vi "Refresh by Name.vi"(6 "TreeControl in":refnum<vi>, 7 "Data Cluster In":T1={"Project"=refnum, "Current Selection"={"Library"=refnum, "VI"=refnum}, "Module ID"=-1, "Tree Selection"=""}, 8 "error in":errorcluster, 11 "Module Name":string) -> (0 "error out":errorcluster, 5 "Data Cluster Out":T1={"Project"=refnum, "Current Selection"={"Library"=refnum, "VI"=refnum}, "Module ID"=-1, "Tree Selection"=""})   [LabVIEW 2020, in "Panther Dashboard.lvlib"]
doc: "Gets the Singleton and Cloneable references and creates a list of each type of DQMH Modules"
uses:
  Panther Dashboard.lvlib
  Module Data--cluster.ctl
  Class/Project/Project.lvclass
  Class/Library/Library.lvclass
  C:/GitClones/PantherDashboard/src/LabVIEW/Panther Dashboard/Class/LabVIEWItem/LabVIEWItem.lvclass
  Class/VI/VI.lvclass
  Class/Project/Project.lvclass/Project.ctl
  Class/LabVIEWItem/LabVIEWItem.lvclass/LabVIEWItem.ctl
  Class/LabVIEWItem/Item Type--enum.ctl
  Class/Library/Library.lvclass/Library.ctl
  Class/Library/Write VIs MAP.vi
  Class/LabVIEWItem/Read Item Name.vi
  Class/Project/Write Libraries.vi
  Class/Project/Read Libraries.vi
  Class/LabVIEWItem/Read Item Tag.vi
  Class/Project/Read Main App Inst Ref.vi
  Class/LabVIEWItem/LabVIEWItem.lvclass
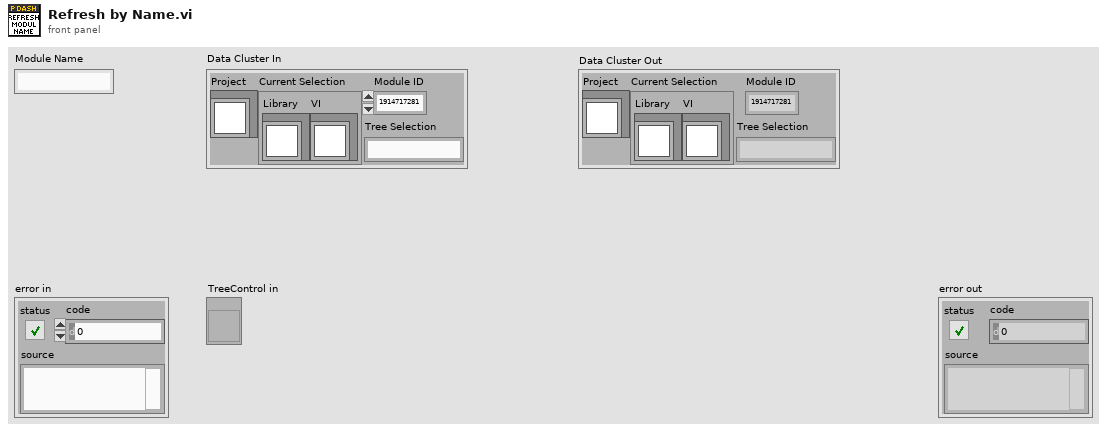
[diagram p1: front panel]
types:
  T1 = typedef "Panther Dashboard.lvlib/Module Data--cluster.ctl" = cluster{"Project":refnum<class "Project.lvclass">, "Current Selection":cluster{"Library":refnum<class "Library.lvclass">, "VI":refnum<class "VI.lvclass">}, "Module ID":i32, "Tree Selection":string}
  T2 = typedef "Panther Dashboard.lvlib/LabVIEWItem.lvclass/Item Type--enum.ctl" = enum16{"Requests", "Broadcasts", "Request and Wait for Reply", "Round Trip", "» Public API VIs", "» Constant VIs", "» Error VIs", "Module", "Project", "No Drag Selection"}
  T3 = typedef "Tree Map.lvlib/Tree Map Data.ctl" = map{string, cluster{"Child Paths Set":set{string}, "Name":string, "Data":string, "Attributes":map{string, string}}}
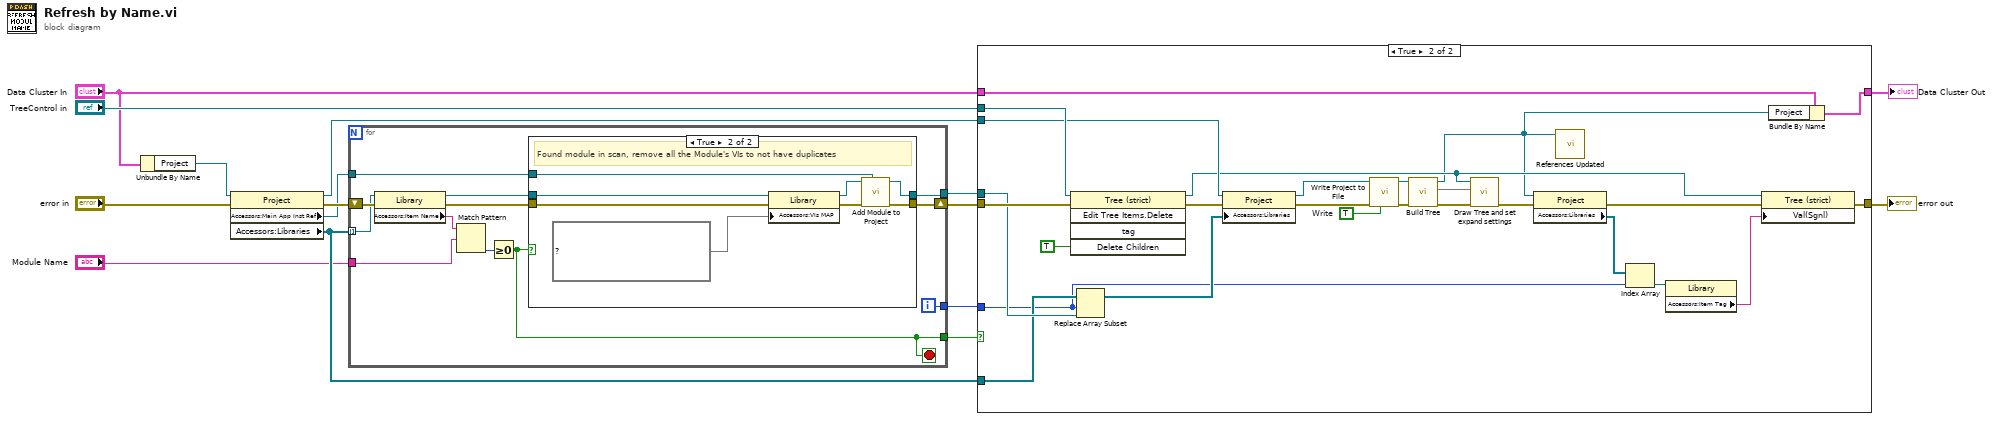
[diagram p0: block diagram]
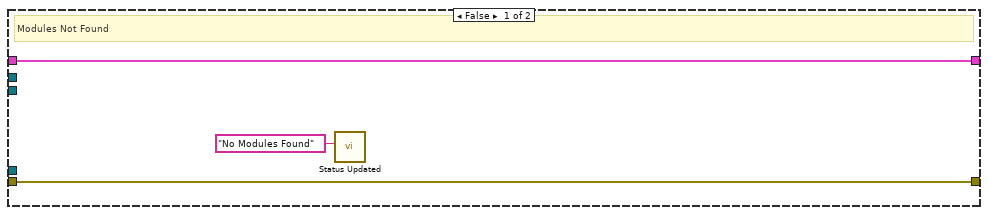
[diagram p2: hidden frame]
diagram:
  n1 = Unbundle By Name("Data Cluster In") -> ("Project"=w8:refnum<class "Project.lvclass">)
  n2 = property class="Project"(reference=w8, error in="error in") -> (reference out=w7:refnum<class "Project.lvclass">, error out=w15:errorcluster, "Accessors:Main App Inst Ref"=w3:refnum<vi>, "Accessors:Libraries"=w4:refnum<class "Library.lvclass">[])
  n3 = for {
    tunnel: w4 -> [w24] mode=indexing
    tunnel: [w23] -> w6
    shift-right: [w25] -> w13
    shift-left: w15 -> [w27]
    tunnel: [w20] -> w5
    tunnel: w3 -> [w21]
    tunnel: "Module Name" -> [w18]
    tunnel: [w16] -> w1
    i -> [w23]
    stop <- w16 stop-if-true
    n4 = property class="Library"(reference=w24, error in=w27) -> (reference out=w22:refnum<class "Library.lvclass">, error out=w26:errorcluster, "Accessors:Item Name"=w19:string)
    n5 = Match Pattern(string=w19, regular expression=w18) -> (offset past match=w17:i32)  [unwired: 1 in, 3 out]
    n6 = Greater Or Equal To 0?(x=w17) -> (x >= 0?=w16:bool)
    n7 = case shown="True" w16 {
      tunnel: w26 -> [w29 w37]
      tunnel: [w29 w36] -> w25
      tunnel: w22 -> [w28 w32]
      tunnel: w21 -> [_ w34]
      tunnel: [w28 w33] -> w20
      frame False {
        # "Current module has different Tag"
      }
      frame True {
        # "Found module in scan, remove all the Module's VIs to not have duplicates"
        n8 = property class="Library"(reference=w32, error in=w37, "Accessors:VIs MAP"=map{T2, refnum<class "VI.lvclass">[]} {} ("VIs MAP")) -> (reference out=w31:refnum<class "Library.lvclass">, error out=w35:errorcluster)
        n9 = call "Add Module to Project.vi"("App Ref"=w34, "error in"=w35, "Library In"=w31) -> ("error out"=w36:errorcluster, "Library Out"=w33:refnum<class "Library.lvclass">)  [unwired: 7 in]
      }
    }
  }
  n10 = case shown="True" w1 {
    tunnel: w13 -> [w40 w66]
    tunnel: [w40 w63] -> w12
    tunnel: "TreeControl in" -> [_ w58]
    tunnel: "Data Cluster In" -> [w39 w55]
    tunnel: [w39 w54] -> w9
    tunnel: w7 -> [_ w53]
    tunnel: w6 -> [_ w44]
    tunnel: w5 -> [_ w49]
    tunnel: w4 -> [_ w46]
    frame False {
      # "Modules Not Found"
      n11 = call "Status Updated.vi"("Status"="No Modules Found") -> ()  [unwired: 10 in, 1 out]
    }
    frame True {
      w56 = TRUE  # Write
      n12 = invoke class="Tree (strict)" method="Edit Tree Items.Delete"(reference=w58, error in=w66, "Delete Children"=TRUE ("Delete Children?")) -> (reference out=w48:refnum<vi>, error out=w65:errorcluster)  [unwired: 2 in, 3 out]
      n13 = Replace Array Subset "Replace Array Subset"(array=w46, new element=w49, index=w44) -> (w47:refnum<class "Library.lvclass">[])
      n14 = property class="Project"(reference=w53, error in=w65, "Accessors:Libraries"=w47) -> (reference out=w51:refnum<class "Project.lvclass">, error out=w62:errorcluster)
      n15 = call "Write Project to File.vi"("Write"=w56, "error in"=w62, "Project In"=w51) -> ("error out"=w61:errorcluster, "Project Out"=w50:refnum<class "Project.lvclass">)  [unwired: 6 in, 1 out]
      n16 = call "Build Tree.vi"("error in"=w61, "Project in"=w50) -> ("error out"=w64:errorcluster, "Tree Map Out"=w52:T3, "Project Out"=w41:refnum<class "Project.lvclass">)  [unwired: 7 in]
      n17 = call "Draw Tree and set expand settings.vi"("error in"=w64, "Tree Map In"=w52, "TreeControl in"=w48) -> ("error out"=w60:errorcluster)  [unwired: 8 in]
      n18 = property class="Project"(reference=w41, error in=w60) -> (error out=w59:errorcluster, "Accessors:Libraries"=w45:refnum<class "Library.lvclass">[])  [unwired: 1 out]
      n19 = call "References Updated.vi"("Project"=w41) -> ()  [unwired: 10 in, 1 out]
      n20 = Index Array(array=w45, index=w44) -> (element=w43:refnum<class "Library.lvclass">)
      n21 = property class="Library"(reference=w43) -> ("Accessors:Item Tag"=w42:string)  [unwired: 1 in, 2 out]
      n22 = property class="Tree (strict)"(reference=w48, error in=w59, "Val(Sgnl)"=w42) -> (error out=w63:errorcluster)  [unwired: 1 out]
      n23 = Bundle By Name(cluster=w55, "Project"=w41) -> (w54:T1)
    }
  }
  "error out" <- w12
  "Data Cluster Out" <- w9
